vi "Stall D open_low.vi"(7 "Port (Port D)":T1=3 items=["Port A", "Port B", "Port C", "Port D"], 9 "Power":i8=30, 11 "NXT/EV3":T2) -> (3 "NXT/EV3":T2)   [LabVIEW 2016]
uses:
  <vilib>/NXT/Subs/LVHSConnector.ctl
  <vilib>/NXT/LegoClasses/BrickReference/BrickReference.lvclass
  <vilib>/NXT/Block Support/NXT_OutputPort.ctl
  <vilib>/NXT/Block Support/NXT_TimerIndex.ctl
  <vilib>/NXT/NXTIO Xnodes/NXTIONodeSubVIs/NXTMoveMotors.vi
  <vilib>/NXT/NXTIO Xnodes/NXTIONodeSubVIs/LEGOResetMotors.vi
  <vilib>/NXT/Dual Mode Library/Sensors/Reset_Timer.vi
  <vilib>/NXT/Dual Mode Library/Waits/Wait_Num.vi
  <vilib>/NXT/Dual Mode Library/Motors/Rotation.vi
  <vilib>/NXT/Dual Mode Library/Sensors/Read_Timer.vi
  <vilib>/NXT/NXTIO Xnodes/NXTIONodeSubVIs/NXTStopMotors.vi
  <vilib>/NXT/NXTIO Xnodes/NXTIOXNode/NXTIO.xnode
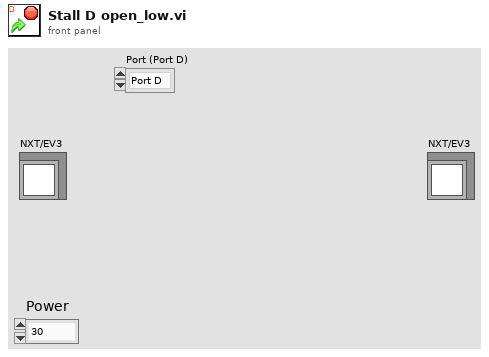
[diagram p1: front panel]
types:
  T1 = typedef "NXT_OutputPort.ctl" = u8
  T2 = typedef "LVHSConnector.ctl" = refnum<class "BrickReference.lvclass">
  T3 = typedef "NXT_TimerIndex.ctl" = u8
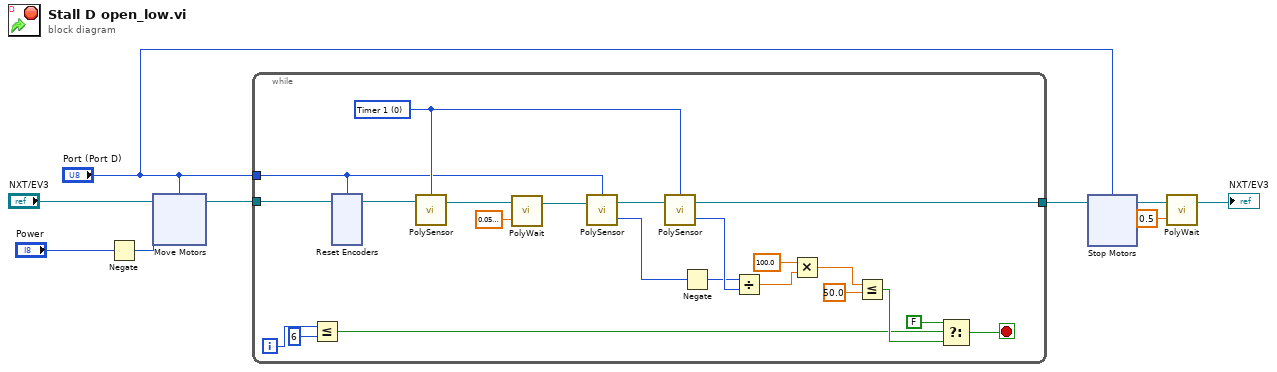
[diagram p0: block diagram]
diagram:
  n1 = Negate(x="Power") -> (-x=w2:i8)
  n2 = xnode "Move Motors"("Power/Speed 1"=w2, "Motors"="Port (Port D)", "NXT/EV3"="NXT/EV3") -> ("NXT/EV3"=w9:T2)
  n3 = while {
    tunnel: w9 -> [w23]
    tunnel: [w22] -> w8
    tunnel: "Port (Port D)" -> [w21]
    i -> [w12]
    stop <- w16 stop-if-true
    w27 = T3 0 items=["Timer 1", "Timer 2", "Timer 3"] ("Timer (Timer 1)")
    n4 = Less Or Equal?(x=w12, y=6) -> (x <= y?=w10:bool)
    n5 = xnode "Reset Encoders"("Motors"=w21, "NXT/EV3"=w23) -> ("NXT/EV3"=w31:T2)
    n6 = call-poly <vilib>:"PolySensor.vi"("NXT/EV3"=w31, "Timer (Timer 1)"=w27) -> ("NXT/EV3"=w30:T2)  [unwired: 2 in]
    n7 = call-poly <vilib>:"PolyWait.vi"("Time (1 sec)"=sgl 0.05, "NXT/EV3"=w30) -> ("NXT/EV3"=w28:T2)  [unwired: 2 in]
    n8 = call-poly <vilib>:"PolySensor.vi"("NXT/EV3"=w28, "Port (Port A)"=w21) -> ("Angle of Rotation"=w25:i32, "NXT/EV3"=w26:T2)  [unwired: 1 in]
    n9 = call-poly <vilib>:"PolySensor.vi"("NXT/EV3"=w26, "Timer (Timer 1)"=w27) -> ("Value (msec)"=w24:u32, "NXT/EV3"=w22:T2)  [unwired: 1 in]
    n10 = Negate(x=w25) -> (-x=w14:i32)
    n11 = Divide(x=w14, y=w24) -> (x/y=w20:dbl)
    n12 = Multiply(x=100.0, y=w20) -> (x*y=w19:dbl)
    n13 = Less Or Equal?(x=w19, y=50.0) -> (x <= y?=w15:bool)
    n14 = Select(t=FALSE, s=w10, f=w15) -> (s? t:f=w16:bool)
  }
  n15 = xnode "Stop Motors"("Motors"="Port (Port D)", "NXT/EV3"=w8) -> ("NXT/EV3"=w5:T2)
  n16 = call-poly <vilib>:"PolyWait.vi"("Time (1 sec)"=sgl 0.5, "NXT/EV3"=w5) -> ("NXT/EV3"=→"NXT/EV3":T2)  [unwired: 2 in]
